vi "Teleop.vi"(10 "Match Info":T1={"Autonomous Elapsed Seconds"=0.0, "TeleOp Elapsed Seconds"=0.0, "Disabled Elapsed Seconds"=0.0, "Visited Autonomous"=FALSE, "Visited TeleOp"=FALSE, "Visited Disabled"=FALSE, "Autonomous Settings"={"Autonomous Style"=enum."Independent", "VI Refnum"=refnum}}, 11 "Call Context":T2) -> ()   [LabVIEW 2018]
doc: "This VI is called for each TeleOp packet received from the DS where the robot is not disabled. It is often used to read from the joysticks and update I/O or to update setpoints for timed control loops. It should complete and return within 20 milliseconds or it may miss DS packets."
uses:
  <vilib>/Rock Robotics/WPI/DriverStation/WPI_DriverStationDerivedRobotMode.ctl
  <vilib>/Rock Robotics/WPI/DriverStation/WPI_DriverStationMatch Info.ctl
  <vilib>/Rock Robotics/WPI/ThirdParty/Phoenix-LabVIEW/Motor Controller/Controls/CTRE_Phoenix_MotorControl_ControlMode.ctl
  <vilib>/Rock Robotics/WPI/Solenoid/WPI_SolenoidValue.ctl
  <vilib>/Rock Robotics/WPI/Utilities/WPI_GetSetVariantRefNum.vi
  <vilib>/Rock Robotics/Network Tables/NT Write Boolean Array.vi
  <vilib>/Rock Robotics/Network Tables/NT Write Numeric Array.vi
  <vilib>/Rock Robotics/Network Tables/NT Read Boolean.vi
  <vilib>/Rock Robotics/Network Tables/NT Read Number.vi
  <vilib>/Rock Robotics/WPI/Solenoid/WPI_SolenoidSetEnum.vi
  <vilib>/Rock Robotics/Network Tables/NT Write Boolean.vi
panel:
  out "Sample Slider 0":dbl(slide) scale=0.0..5.0
  out "Sample Boolean 1":bool
  out "Sample Boolean 0":bool
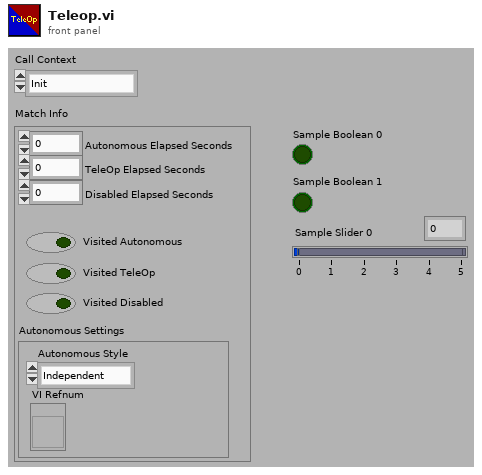
[diagram p1: front panel]
types:
  T1 = typedef "WPI_DriverStationMatch Info.ctl" = cluster{"Autonomous Elapsed Seconds":dbl, "TeleOp Elapsed Seconds":dbl, "Disabled Elapsed Seconds":dbl, "Visited Autonomous":bool, "Visited TeleOp":bool, "Visited Disabled":bool, "Autonomous Settings":cluster{"Autonomous Style":enum16{"Iterative", "Independent"}, "VI Refnum":refnum<vi>}}
  T2 = typedef "WPI_DriverStationDerivedRobotMode.ctl" = enum16{"Init", "Execute", "Stop"}
  T3 = typedef "CTRE_Phoenix_MotorControl_ControlMode.ctl" = u16
  T4 = typedef "WPI_JoystickDevRef.ctl" = cluster{"Device":T5}
  T5 = typedef "WPI_JoystickDeviceEnum.ctl" = enum16{"USB 0", "USB 1", "USB 2", "USB 3", "USB 4", "USB 5"}
  T6 = typedef "WPI_SolenoidValue.ctl" = enum16{"Off", "On", "Forward", "Reverse"}
  T7 = typedef "WPI_SolenoidDevRef.ctl" = cluster{"DevStatus":errorcluster, "Pneumatics Control Module":u8, "Forward Solenoid Channel":T8, "Reverse Solenoid Channel":T8}
  T8 = typedef "WPI_SolenoidChannel.ctl" = enum8{"Solenoid 0", "Solenoid 1", "Solenoid 2", "Solenoid 3", "Solenoid 4", "Solenoid 5", "Solenoid 6", "Solenoid 7", "Invalid"}
  T9 = typedef "WPI_MotorControlDeviceRef.ctl" = cluster{"DeviceStatus":errorcluster, "Type":T10, "PWM":cluster{"PWM Channel":T11, "DeadBand":T12}, "CAN":cluster{"Device Number":u8, "SetOutput VI Ref":variant, "GetOutput VI Ref":variant, "Enable VI Ref":variant, "Disable VI Ref":variant, "Data":variant}, "Invert":bool, "DIO PWM":cluster{"PWM \"Enable\" Channel":T11, "DIOChannel":T13, "PWM Rate":dbl}}
  T10 = typedef "WPI_MotorControlType.ctl" = enum16{"PWM", "CAN", "DIO PWM"}
  T11 = typedef "FPGA_DIOPWMChannel.ctl" = enum8{"PWM 0", "PWM 1", "PWM 2", "PWM 3", "PWM 4", "PWM 5", "PWM 6", "PWM 7", "PWM 8", "PWM 9", "PWM MXP 0", "PWM MXP 1", "PWM MXP 2", "PWM MXP 3", "PWM MXP 4", "PWM MXP 5", "PWM MXP 6", "PWM MXP 7", "PWM MXP 8", "PWM MXP 9", "Invalid"}
  T12 = typedef "WPI_PWMDeadband.ctl" = cluster{"Name":string, "maxPositivePwm":i32, "minPositivePwm":i32, "centerPwm":i32, "maxNegativePwm":i32, "minNegativePwm":i32, "angularRange":u16}
  T13 = typedef "FPGA_DIOChannel.ctl" = enum8{"DIO 0", "DIO 1", "DIO 2", "DIO 3", "DIO 4", "DIO 5", "DIO 6", "DIO 7", "DIO 8", "DIO 9", "DIO MXP 0", "DIO MXP 1", "DIO MXP 2", "DIO MXP 3", "DIO MXP 4", "DIO MXP 5", "DIO MXP 6", "DIO MXP 7", "DIO MXP 8", "DIO MXP 9", "DIO MXP 10", "DIO MXP 11", "DIO MXP 12", "DIO MXP 13", "DIO MXP 14", "DIO MXP 15", "SPI Port CS1", "SPI Port CS2", "SPI Port CS3", "SPI Port MISO", "SPI Port MOSI", "Invalid"}
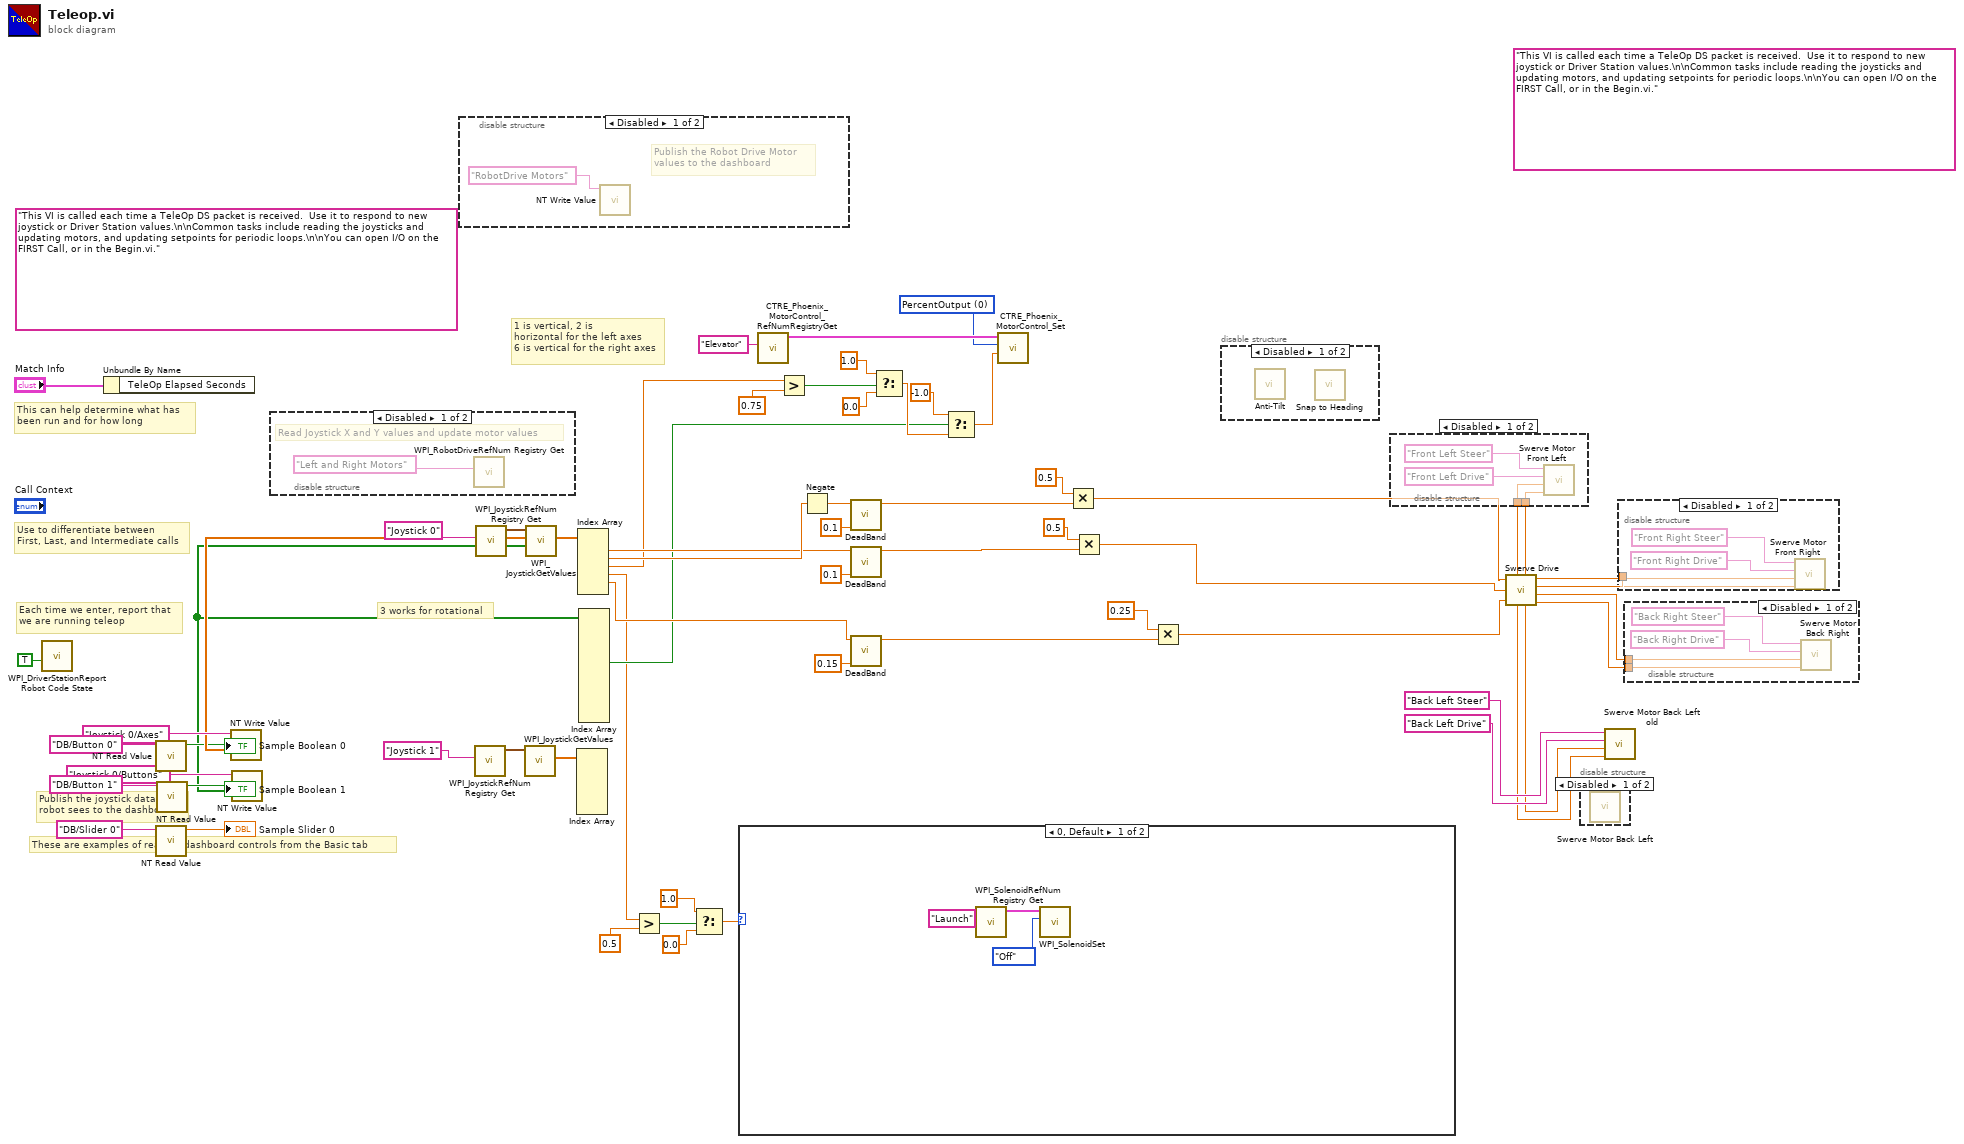
[diagram p0: block diagram]
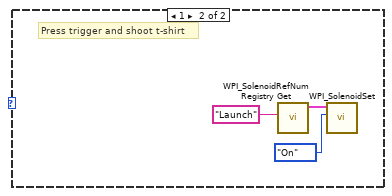
[diagram p9: hidden frame]
diagram:
  w34 = T3 0 items=["PercentOutput"=0, "Position"=1, "Velocity"=2, "Current"=3, "Follower"=5, "MotionProfile"=6, "MotionMagic"=7, "MotionMagicArc"=8, "MotionProfileArc"=10, "Disabled"=15] ("Control Mode")
  (unwired) "This VI is called each time a TeleOp DS packet is received.  Use it to respond to new joystick or Driver Station values.\n\nCommon tasks include reading the joysticks and updating motors, and updating setpoints for periodic loops.\n\nYou can open I/O on the FIRST Call, or in the Begin.vi."
  (unwired) "This VI is called each time a TeleOp DS packet is received.  Use it to respond to new joystick or Driver Station values.\n\nCommon tasks include reading the joysticks and updating motors, and updating setpoints for periodic loops.\n\nYou can open I/O on the FIRST Call, or in the Begin.vi."
  # "3 works for rotational"
  # "1 is vertical, 2 is \nhorizontal for the left axes\n6 is vertical for the right axes"
  # "These are examples of reading dashboard controls from the Basic tab"
  # "Publish the joystick data the\nrobot sees to the dashboard"
  # "Each time we enter, report that\nwe are running teleop"
  # "Use to differentiate between\nFirst, Last, and Intermediate calls"
  # "This can help determine what has\nbeen run and for how long"
  n1 = call <vilib>:"WPI_DriverStationReport Robot Code State.vi"("TeleOp"=TRUE ("Autonomous")) -> ()  [unwired: 10 in, 1 out]
  n2 = Unbundle By Name("Match Info") -> ()  [unwired: 1 out]
  n3 = call-poly <vilib>:"NT Read Value.vi"("Name"="DB/Button 0" ("refnum name")) -> ("Boolean"=→"Sample Boolean 0":bool)  [unwired: 9 in, 1 out]
  n4 = call-poly <vilib>:"NT Read Value.vi"("Name"="DB/Slider 0" ("refnum name")) -> ("Numeric"=→"Sample Slider 0":dbl)  [unwired: 9 in, 1 out]
  n5 = call-poly <vilib>:"NT Read Value.vi"("Name"="DB/Button 1" ("refnum name")) -> ("Boolean"=→"Sample Boolean 1":bool)  [unwired: 9 in, 1 out]
  n6 = disable-structure shown="Disabled" {
    frame Disabled {
      # "Read Joystick X and Y values and update motor values"
      n7 = call <vilib>:"WPI_RobotDriveRefNum Registry Get.vi"("refnum name"="Left and Right Motors") -> ()  [unwired: 1 in, 10 out]
    }
    frame Enabled {
    }
  }
  n8 = disable-structure shown="Disabled" {
    frame Disabled {
      # "Publish the Robot Drive Motor\nvalues to the dashboard"
      n9 = call-poly <vilib>:"NT Write Value.vi"("Name"="RobotDrive Motors") -> ()  [unwired: 10 in, 1 out]
    }
    frame Enabled {
    }
  }
  n10 = call <vilib>:"WPI_JoystickRefNum Registry Get.vi"("refnum name"="Joystick 1") -> ("JoystickDevRef"=w41:T4)  [unwired: 1 in, 9 out]
  n11 = call <vilib>:"WPI_JoystickRefNum Registry Get.vi"("refnum name"="Joystick 0") -> ("JoystickDevRef"=w59:T4)  [unwired: 1 in, 9 out]
  n12 = call <vilib>:"WPI_JoystickGetValues.vi"("JoystickDevRef"=w41) -> ("Axes"=w40:dbl[])  [unwired: 6 in, 4 out]
  n13 = call <vilib>:"WPI_JoystickGetValues.vi"("JoystickDevRef"=w59) -> ("Buttons"=w48:bool[], "Axes"=w55:dbl[])  [unwired: 6 in, 3 out]
  n14 = call-poly <vilib>:"NT Write Value.vi"("Numeric Array"=w55, "Name"="Joystick 0/Axes") -> ()  [unwired: 9 in, 1 out]
  n15 = call-poly <vilib>:"NT Write Value.vi"("Boolean Array"=w48, "Name"="Joystick 0/Buttons") -> ()  [unwired: 9 in, 1 out]
  n16 = Index Array(array=w40) -> ()  [unwired: 6 in, 6 out]
  n17 = Index Array(array=w55) -> (element #1=w45:dbl, element #2=w47:dbl, element #3=w26:dbl, element #4=w19:dbl, element #5=w29:dbl)  [unwired: 6 in, 1 out]
  n18 = Index Array(array=w48) -> (element #5=w28:bool)  [unwired: 12 in, 11 out]
  n19 = Greater?(x=w19, y=0.5 ("f")) -> (0:w22:bool)
  n20 = Select(t=1.0, s=w22, f=0.0) -> (s? t:f=w18:dbl)
  n21 = case shown="0, Default" w18 {
    frame 0, Default {
      n22 = call <vilib>:"WPI_SolenoidRefNum Registry Get.vi"("refnum name"="Launch") -> ("SolenoidDevRef"=w65:T7)  [unwired: 9 in, 1 out]
      n23 = call-poly <vilib>:"WPI_SolenoidSet.vi"("Value"=WPI_SolenoidValue."Off", "SolenoidDevRef"=w65) -> ()  [unwired: 8 in, 2 out]
    }
    frame 1 {
      # "Press trigger and shoot t-shirt"
      n24 = call <vilib>:"WPI_SolenoidRefNum Registry Get.vi"("refnum name"="Launch") -> ("SolenoidDevRef"=w69:T7)  [unwired: 9 in, 1 out]
      n25 = call-poly <vilib>:"WPI_SolenoidSet.vi"("Value"=WPI_SolenoidValue."On", "SolenoidDevRef"=w69) -> ()  [unwired: 8 in, 2 out]
    }
  }
  n26 = call <vilib>:"CTRE_Phoenix_MotorControl_RefNumRegistryGet.vi"("refnum name"="Elevator") -> ("PhoenixMotorControlDevRef"=w35:T9)  [unwired: 9 in, 1 out]
  n27 = Greater?(x=w26, y=0.75 ("f")) -> (0:w25:bool)
  n28 = Negate(x=w47) -> (-x=w46:dbl)
  n29 = call "DeadBand.vi"("Deadband"=0.1, "Input"=w46) -> ("Output"=w17:dbl)  [unwired: 9 in]
  n30 = call "DeadBand.vi"("Deadband"=0.1, "Input"=w45) -> ("Output"=w15:dbl)  [unwired: 9 in]
  n31 = call "DeadBand.vi"("Deadband"=0.15, "Input"=w29) -> ("Output"=w38:dbl)  [unwired: 9 in]
  n32 = Select(t=1.0, s=w25, f=0.0) -> (s? t:f=w32:dbl)
  n33 = Select(t=-1.0, s=w28, f=w32) -> (s? t:f=w30:dbl)
  n34 = call <vilib>:"CTRE_Phoenix_MotorControl_Set.vi"("Output"=w30, "Control Mode"=w34, "PhoenixMotorControlDevRef"=w35) -> ()  [unwired: 7 in, 2 out]
  n35 = Multiply(x=0.5, y=w17) -> (x*y=w16:dbl)
  n36 = Multiply(x=0.5 ("y"), y=w15) -> (x*y=w14:dbl)
  n37 = Multiply(x=0.25 ("y"), y=w38) -> (x*y=w37:dbl)
  n38 = disable-structure shown="Disabled" {
    frame Disabled {
      n39 = call "Anti-Tilt.vi"() -> ()  [unwired: 10 in, 2 out]
      n40 = call "Snap to Heading.vi"() -> ()  [unwired: 11 in, 1 out]
    }
    frame Enabled {
    }
  }
  n41 = call "Swerve Drive.vi"("Longitudinal - Y"=w16, "Lateral - X"=w14, "Rotational - Z"=w37) -> ("Front Left Speed"=w6:dbl, "Back Left Angle"=w1:dbl, "Front Left Angle"=w5:dbl, "Front Right Speed"=w7:dbl, "Front Right Angle"=w8:dbl, "Back Left Speed"=w2:dbl, "Back Right Speed"=w10:dbl, "Back Right Angle"=w9:dbl)
  n42 = disable-structure shown="Disabled" {
    disable-tunnel: w6 -> [w73 _]
    disable-tunnel: w5 -> [w72 _]
    frame Disabled {
      n43 = call "Swerve Motor Front Left.vi"("Steer motor reference name"="Front Left Steer", "Drive motor reference name"="Front Left Drive", "Speed command"=w73, "Direction command (deg)"=w72) -> ()  [unwired: 6 in]
    }
    frame Enabled {
    }
  }
  n44 = disable-structure shown="Disabled" {
    frame Disabled {
      n45 = call "Swerve Motor Back Left.vi"() -> ()  [unwired: 10 in]
    }
    frame Enabled {
    }
  }
  n46 = call "Swerve Motor Back Left old.vi"("Steer motor reference name"="Back Left Steer", "Drive motor reference name"="Back Left Drive", "Speed command"=w2, "Direction command (deg)"=w1) -> ()  [unwired: 6 in]
  n47 = disable-structure shown="Disabled" {
    disable-tunnel: w8 -> [w77 _]
    disable-tunnel: w7 -> [w76 _]
    frame Disabled {
      n48 = call "Swerve Motor Front Right.vi"("Steer motor reference name"="Front Right Steer", "Drive motor reference name"="Front Right Drive", "Speed command"=w76, "Direction command (deg)"=w77) -> ()  [unwired: 6 in]
    }
    frame Enabled {
    }
  }
  n49 = disable-structure shown="Disabled" {
    disable-tunnel: w10 -> [w81 _]
    disable-tunnel: w9 -> [w80 _]
    frame Disabled {
      n50 = call "Swerve Motor Back Right.vi"("Steer motor reference name"="Back Right Steer", "Drive motor reference name"="Back Right Drive", "Speed command"=w81, "Direction command (deg)"=w80) -> ()  [unwired: 6 in]
    }
    frame Enabled {
    }
  }
